vi "ParseLakeshoreSettings (SubVI).vi"(0 "Settings array in":i32[](array[numeric])) -> (1 "Array":string[](array[string]), 2 "Current excitation (A)":dbl)   [LabVIEW 2017, in "Fridge Software v2.1.lvlib"]
uses:
  Fridge Software v2.1.lvlib
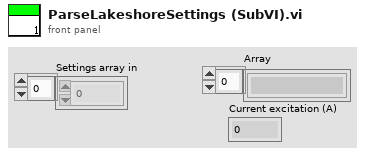
[diagram p1: front panel]
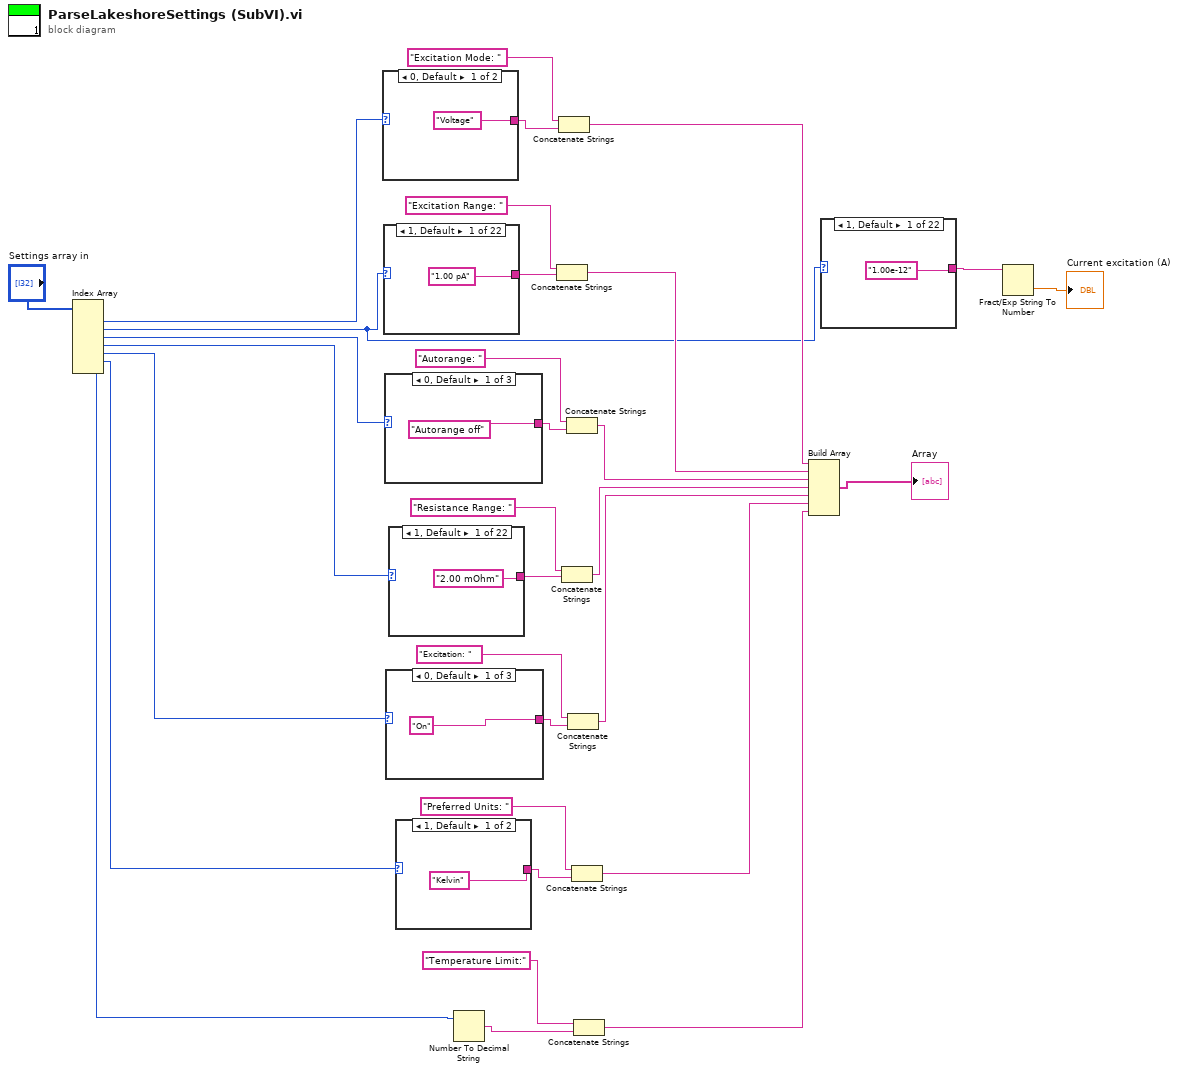
[diagram p0: block diagram]
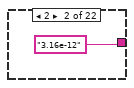
[diagram p2: hidden frame]
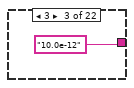
[diagram p3: hidden frame]
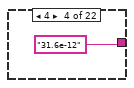
[diagram p4: hidden frame]
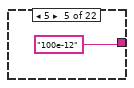
[diagram p5: hidden frame]
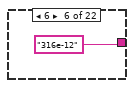
[diagram p6: hidden frame]
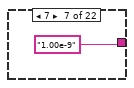
[diagram p7: hidden frame]
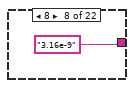
[diagram p8: hidden frame]
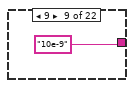
[diagram p9: hidden frame]
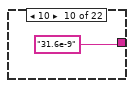
[diagram p10: hidden frame]
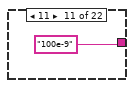
[diagram p11: hidden frame]
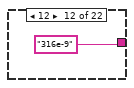
[diagram p12: hidden frame]
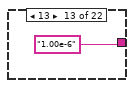
[diagram p13: hidden frame]
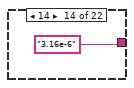
[diagram p14: hidden frame]
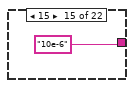
[diagram p15: hidden frame]
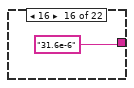
[diagram p16: hidden frame]
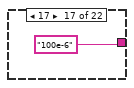
[diagram p17: hidden frame]
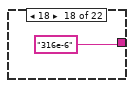
[diagram p18: hidden frame]
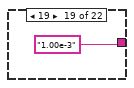
[diagram p19: hidden frame]
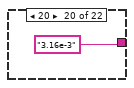
[diagram p20: hidden frame]
diagram:
  n1 = Index Array(array="Settings array in") -> (element #1=w31:i32, element #2=w3:i32, element #3=w30:i32, element #4=w18:i32, element #5=w12:i32, element #6=w16:i32, element #7=w15:i32)  [unwired: 7 in]
  n2 = case shown="0, Default" w31 {
    tunnel: ["Voltage" "Current"] -> w28
    frame 0, Default {
    }
    frame 1 {
    }
  }
  n3 = case shown="1, Default" w3 {
    tunnel: ["1.00 pA" "3.16 pA" "10.0 pA" "31.6 pA" "100 pA" "316 pA" "1.00 nA" "3.16 nA" "10 nA" "31.6 nA" "100 nA" "316 nA" "1.00 uA" "3.16 uA" "10 uA" "31.6 uA" "100 uA" "316 uA" "1.00 mA" "3.16 mA" "10 mA" "31.6 mA"] -> w26
    frame 1, Default {
    }
    frame 2 {
    }
    frame 3 {
    }
    frame 4 {
    }
    frame 5 {
    }
    frame 6 {
    }
    frame 7 {
    }
    frame 8 {
    }
    frame 9 {
    }
    frame 10 {
    }
    frame 11 {
    }
    frame 12 {
    }
    frame 13 {
    }
    frame 14 {
    }
    frame 15 {
    }
    frame 16 {
    }
    frame 17 {
    }
    frame 18 {
    }
    frame 19 {
    }
    frame 20 {
    }
    frame 21 {
    }
    frame 22 {
    }
  }
  n4 = case shown="0, Default" w30 {
    tunnel: ["Autorange off" "Autorange Current" "ROX 102B Autorange"] -> w24
    frame 0, Default {
    }
    frame 1 {
    }
    frame 2 {
    }
  }
  n5 = case shown="0, Default" w12 {
    tunnel: ["On" "Off" "ROX 102B Autorange"] -> w13
    frame 0, Default {
    }
    frame 1 {
    }
    frame 2 {
    }
  }
  n6 = case shown="1, Default" w18 {
    tunnel: ["2.00 mOhm" "6.32 mOhm" "20.0 mOhm" "63.2 mOhm" "200 mOhm" "632 mOhm" "2.00 Ohm" "6.32 Ohm" "20.0 Ohm" "63.2 Ohm" "200 Ohm" "632 Ohm" "2.00 kOhm" "6.32 kOhm" "20.0 kOhm" "63.2 kOhm" "200 kOhm" "632 kOhm" "2 MOhm" "6.32 MOhm" "20 MOhm" "63.2 MOhm"] -> w22
    frame 1, Default {
    }
    frame 2 {
    }
    frame 3 {
    }
    frame 4 {
    }
    frame 5 {
    }
    frame 6 {
    }
    frame 7 {
    }
    frame 8 {
    }
    frame 9 {
    }
    frame 10 {
    }
    frame 11 {
    }
    frame 12 {
    }
    frame 13 {
    }
    frame 14 {
    }
    frame 15 {
    }
    frame 16 {
    }
    frame 17 {
    }
    frame 18 {
    }
    frame 19 {
    }
    frame 20 {
    }
    frame 21 {
    }
    frame 22 {
    }
  }
  n7 = case shown="1, Default" w16 {
    tunnel: ["Kelvin" "Ohms"] -> w21
    frame 1, Default {
    }
    frame 2 {
    }
  }
  n8 = Number To Decimal String(number=w15) -> (decimal integer string=w17:string)  [unwired: 1 in]
  n9 = Concatenate Strings("Excitation Range: ", w26) -> (w10:string)
  n10 = Concatenate Strings("Excitation Mode: ", w28) -> (w11:string)
  n11 = Concatenate Strings("Resistance Range: ", w22) -> (w8:string)
  n12 = Concatenate Strings("Autorange: ", w24) -> (w9:string)
  n13 = Concatenate Strings("Excitation: ", w13) -> (w7:string)
  n14 = Concatenate Strings("Preferred Units: ", w21) -> (w6:string)
  n15 = Concatenate Strings("Temperature Limit:", w17) -> (w5:string)
  n16 = Build Array(w11, w10, w9, w8, w7, w6, w5) -> (→"Array":string[])
  n17 = case shown="1, Default" w3 {
    tunnel: ["1.00e-12" "3.16e-12" "10.0e-12" "31.6e-12" "100e-12" "316e-12" "1.00e-9" "3.16e-9" "10e-9" "31.6e-9" "100e-9" "316e-9" "1.00e-6" "3.16e-6" "10e-6" "31.6e-6" "100e-6" "316e-6" "1.00e-3" "3.16e-3" "10e-3" "31.6e-3"] -> w2
    frame 1, Default {
    }
    frame 2 {
    }
    frame 3 {
    }
    frame 4 {
    }
    frame 5 {
    }
    frame 6 {
    }
    frame 7 {
    }
    frame 8 {
    }
    frame 9 {
    }
    frame 10 {
    }
    frame 11 {
    }
    frame 12 {
    }
    frame 13 {
    }
    frame 14 {
    }
    frame 15 {
    }
    frame 16 {
    }
    frame 17 {
    }
    frame 18 {
    }
    frame 19 {
    }
    frame 20 {
    }
    frame 21 {
    }
    frame 22 {
    }
  }
  n18 = Fract/Exp String To Number(string=w2) -> (number=→"Current excitation (A)":dbl)  [unwired: 3 in, 1 out]
